vi "Angular Position.vi"() -> ()   [LabVIEW 2019]
uses:
  Trigger State.ctl
panel:
  out "error IO":errorcluster
  out "Position vs Trigger":cluster{dbl[], dbl[]}[](graph)
  in  "Stop Button":bool
  out "Gauge":dbl(knob) scale=-180.0..180.0
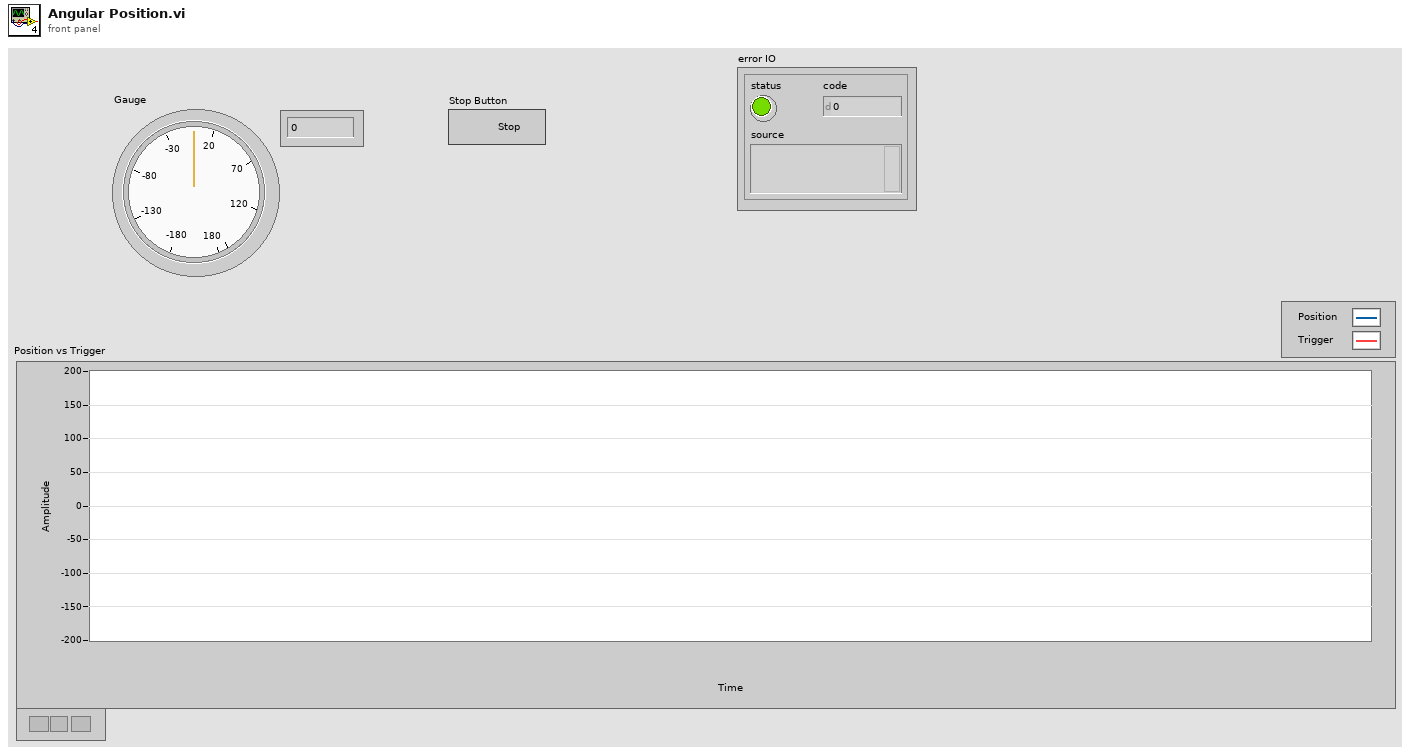
[diagram p1: front panel]
types:
  T1 = typedef "Trigger State.ctl" = enum16{"Below Threshold?", "At or Above Threshold?", "Send Trigger"}
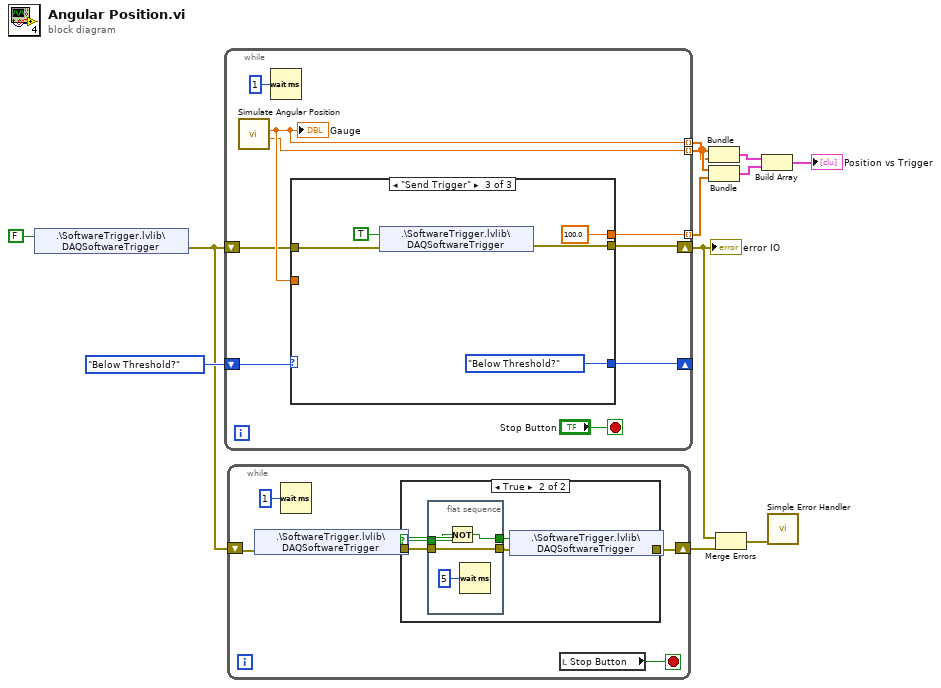
[diagram p0: block diagram]
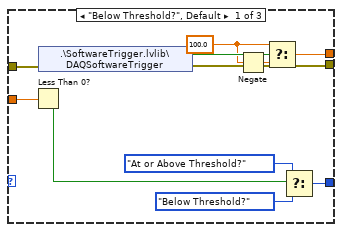
[diagram p3: hidden frame]
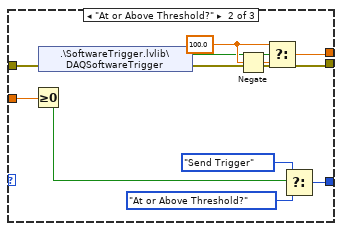
[diagram p4: hidden frame]
diagram:
  n1 = shared-variable ".\\SoftwareTrigger.lvlib\\DAQSoftwareTrigger"(FALSE ("Software Trigger")) -> (error out=w4:errorcluster)  [unwired: 1 in]
  n2 = while {
    shift-right: [w18] -> _
    shift-left: Trigger_State."Below Threshold?" -> [w19]
    tunnel: [w13] -> w8 mode=indexing
    tunnel: [w17] -> w6 mode=indexing
    tunnel: [w16] -> w7 mode=indexing
    shift-right: [w14] -> w3
    shift-left: w4 -> [w15]
    stop <- "Stop Button" stop-if-true
    n3 = call "Simulate Angular Position.vi"() -> ("Present (s)"=w16:dbl, "Gauge"=w17:dbl)  [unwired: 10 in]
    "Gauge" <- w17
    n4 = Wait (ms)(milliseconds to wait=u32 1) -> ()  [unwired: 1 out]
    n5 = case shown="\"Send Trigger\"" w19 {
      tunnel: w17 -> [w32 w43 _]
      tunnel: [w28 w39 Trigger_State."Below Threshold?" ("t")] -> w18
      tunnel: w15 -> [w26 w36 w46]
      tunnel: [w22 w34 w45] -> w14
      tunnel: [w23 w35 100.0] -> w13
      frame "Below Threshold?", Default {
        w24 = 100.0
        n6 = Less Than 0?(x=w32) -> (x < 0?=w31:bool)
        n7 = shared-variable ".\\SoftwareTrigger.lvlib\\DAQSoftwareTrigger"(error in=w26) -> (w27:bool, error out=w22:errorcluster)
        n8 = Negate(x=w24) -> (-x=w25:dbl)
        n9 = Select(t=w24, s=w27, f=w25) -> (s? t:f=w23:dbl)
        n10 = Select(t=Trigger_State."At or Above Threshold?", s=w31, f=Trigger_State."Below Threshold?") -> (s? t:f=w28:T1)
      }
      frame "At or Above Threshold?" {
        w37 = 100.0
        n11 = Greater Or Equal To 0?(x=w43) -> (x >= 0?=w42:bool)
        n12 = shared-variable ".\\SoftwareTrigger.lvlib\\DAQSoftwareTrigger"(error in=w36) -> (w33:bool, error out=w34:errorcluster)
        n13 = Negate(x=w37) -> (-x=w38:dbl)
        n14 = Select(t=w37, s=w33, f=w38) -> (s? t:f=w35:dbl)
        n15 = Select(t=Trigger_State."Send Trigger", s=w42, f=Trigger_State."At or Above Threshold?") -> (s? t:f=w39:T1)
      }
      frame "Send Trigger" {
        n16 = shared-variable ".\\SoftwareTrigger.lvlib\\DAQSoftwareTrigger"(TRUE ("Software Trigger"), error in=w46) -> (error out=w45:errorcluster)
      }
    }
  }
  "error IO" <- w3
  n17 = while {
    shift-right: [w50] -> w2
    shift-left: w4 -> [w53]
    stop <- w49 stop-if-true
    n18 = shared-variable ".\\SoftwareTrigger.lvlib\\DAQSoftwareTrigger"(error in=w53) -> (w52:bool, error out=w51:errorcluster)
    n19 = Wait (ms)(milliseconds to wait=u32 1) -> ()  [unwired: 1 out]
    n20 = case shown="True" w52 {
      selector: w52 -> [_ w57]
      tunnel: w51 -> [w55 w60]
      tunnel: [w55 w58] -> w50
      frame False {
      }
      frame True {
        n21 = flat-sequence {
          tunnel: w60 -> [w64]
          tunnel: [w64] -> w59
          tunnel: w57 -> [w62]
          tunnel: [w61] -> w56
          frame #0 {
            n22 = Not(x=w62) -> (.not. x?=w61:bool)
            n23 = Wait (ms)(milliseconds to wait=u32 5) -> ()  [unwired: 1 out]
          }
        }
        n24 = shared-variable ".\\SoftwareTrigger.lvlib\\DAQSoftwareTrigger"(w56, error in=w59) -> (error out=w58:errorcluster)
      }
    }
    n25 = local read "Stop Button"() -> (w49:bool)
  }
  n26 = Bundle(w7, w6) -> (w9:cluster{dbl[], dbl[]})  [unwired: 1 in]
  n27 = Bundle(w7, w8) -> (w11:cluster{dbl[], dbl[]})  [unwired: 1 in]
  n28 = Merge Errors(w3, w2) -> (w1:errorcluster)
  n29 = Build Array(w9, w11) -> (→"Position vs Trigger":cluster{dbl[], dbl[]}[])
  n30 = call <vilib>:"Simple Error Handler.vi"("error in (no error)"=w1) -> ()  [unwired: 4 in, 5 out]
